vi "SubVI.vi"(0 "AO0波形参数":T1={"波形类型"=2, "幅值"=1.0, "偏置"=0.0, "占空比"=50.0} {"占空比" format="%0.2p"; "偏置" format="%0.2p"; "幅值" format="%0.2p"; "波形类型" items=["正弦波", "三角波", "方波", "锯齿波"]}, 1 "频率比例系数":dbl=9.0 format="%#_13g", 2 "AO8波形参数":cluster{"方向1电压":dbl, "方向2电压":dbl, "方向3电压":dbl}={"方向1电压"=0.5, "方向2电压"=1.0, "方向3电压"=2.0} {"方向3电压" format="%0.2p"; "方向2电压" format="%0.2p"; "方向1电压" format="%0.2p"}, 5 "AO2波形参数":T3={"波形类型"=2, "幅值"=1.0, "偏置"=0.0, "占空比"=50.0, "周期"=0.025} {"占空比" format="%0.2p"; "偏置" format="%0.2p"; "周期" format="%0.2p"; "幅值" format="%0.2p"; "波形类型" items=["正弦波", "三角波", "方波", "锯齿波"]}, 7 "AO4波形参数":T2={"扫描范围(μm)"=10.0, "步长(μm)"=1.0, "转换系数(V/μm)"=0.5, "等待时间(ms)"=3.0} {"等待时间(ms)" format="%0.2p"; "转换系数(V/μm)" format="%0.2p"; "步长(μm)" format="%0.2p"; "扫描范围(μm)" format="%0.2p"}, 9 "AO6波形参数":T1={"波形类型"=2, "幅值"=1.0, "偏置"=0.0, "占空比"=50.0} {"占空比" format="%0.2p"; "偏置" format="%0.2p"; "幅值" format="%0.2p"; "波形类型" items=["正弦波", "三角波", "方波", "锯齿波"]}, 11 "Error in":errorcluster caption="错误输入（无错误）", 12 "采样率":dbl=10000.0) -> (4 "AO0":waveform(dbl)(graph), 6 "AO2":waveform(dbl)(graph), 8 "AO4":waveform(dbl)(graph), 10 "AO6":waveform(dbl)(graph), 13 "AO8":waveform(dbl)(graph), 14 "采样数":dbl=1000.0, 15 "Error out":errorcluster caption="错误输出")   [LabVIEW 2017]
uses:
  <vilib>/measure/NI_MABase.lvlib
  <vilib>/Analysis/NI_AALBase.lvlib
  <vilib>/Analysis/baseanly.llb/Mean (DBL).vi
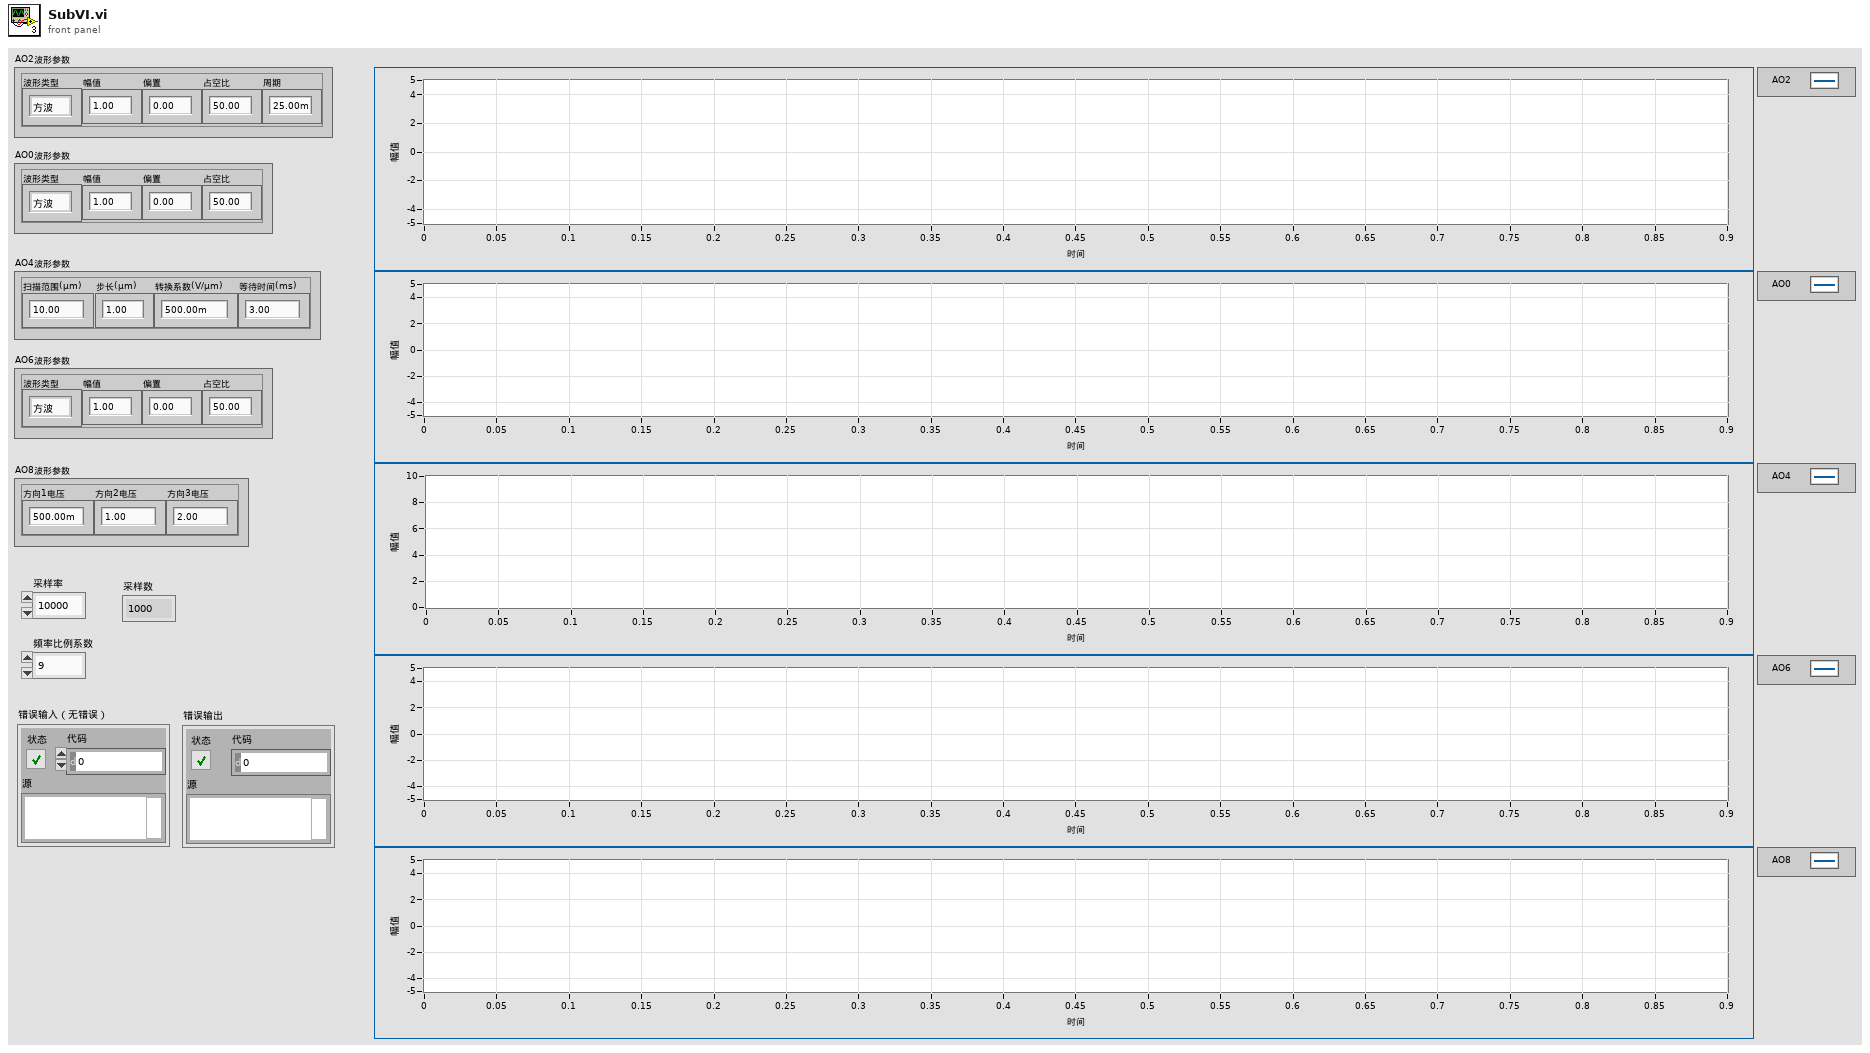
[diagram p1: front panel]
types:
  T1 = cluster{"波形类型":u16, "幅值":dbl, "偏置":dbl, "占空比":dbl}
  T2 = cluster{"扫描范围(μm)":dbl, "步长(μm)":dbl, "转换系数(V/μm)":dbl, "等待时间(ms)":dbl}
  T3 = cluster{"波形类型":u16, "幅值":dbl, "偏置":dbl, "占空比":dbl, "周期":dbl}
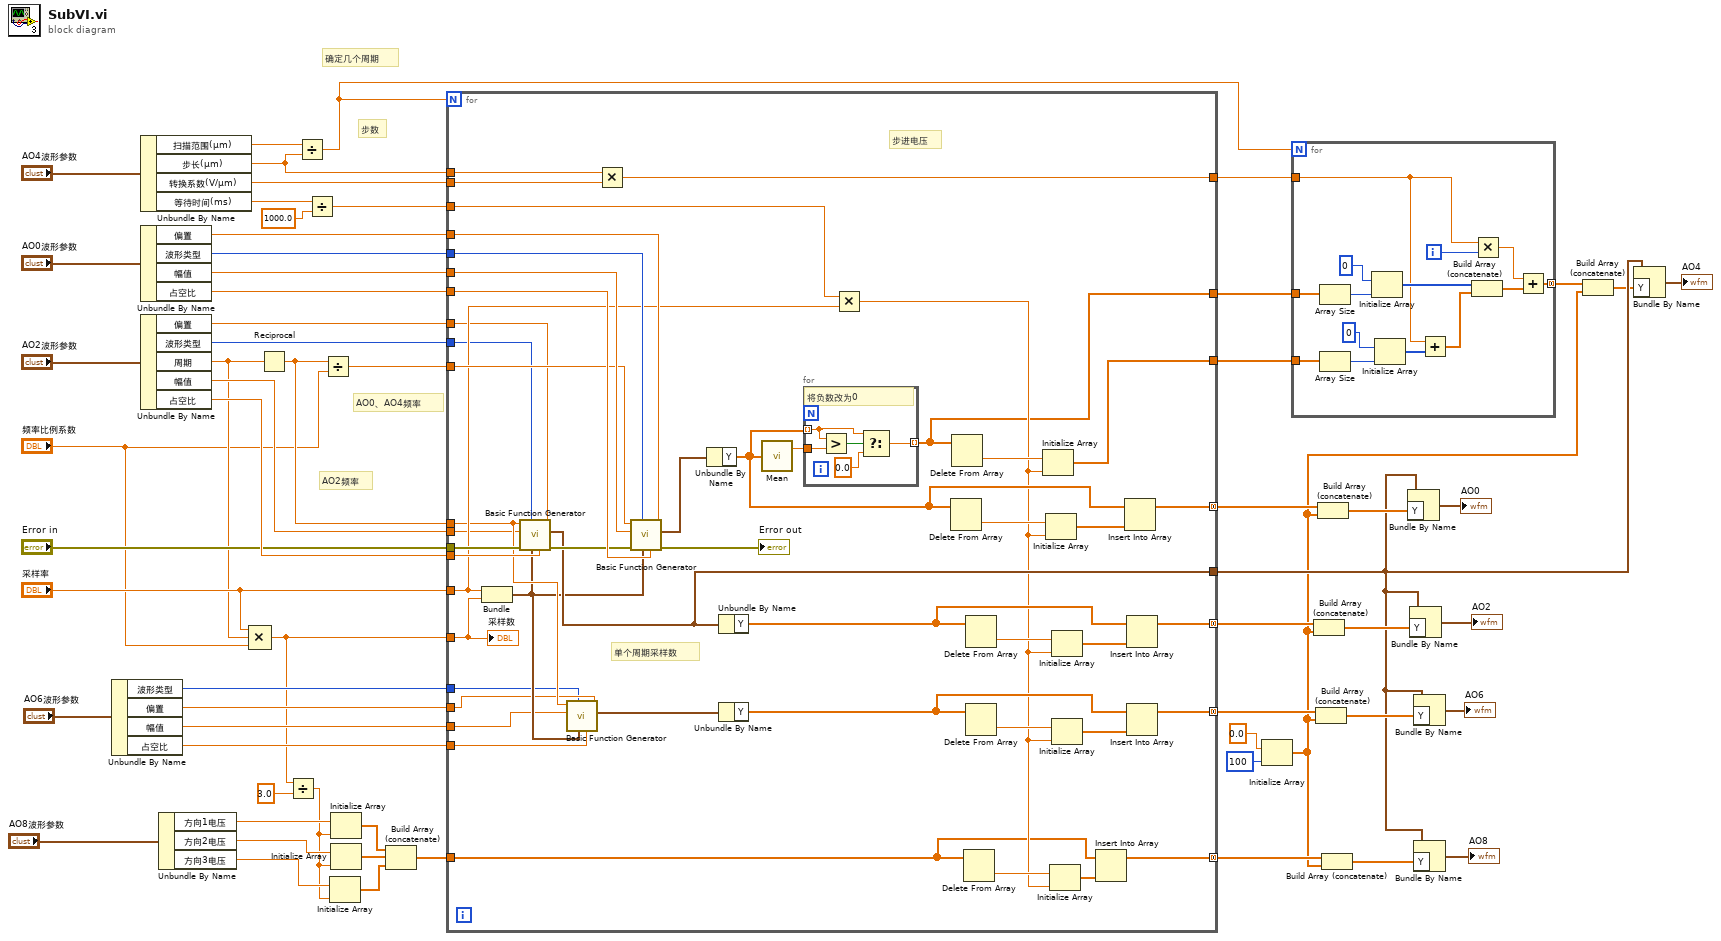
[diagram p0: block diagram]
diagram:
  # "步数"
  # "AO2频率"
  # "AO0、AO4频率"
  # "确定几个周期"
  n1 = Unbundle By Name("AO6波形参数") -> ("波形类型"=w33:u16, "偏置"=w34:dbl, "幅值"=w35:dbl, "占空比"=w36:dbl)
  n2 = Unbundle By Name("AO4波形参数") -> ("扫描范围(μm)"=w49:dbl, "步长(μm)"=w50:dbl, "转换系数(V/μm)"=w51:dbl, "等待时间(ms)"=w46:dbl)
  n3 = Unbundle By Name("AO0波形参数") -> ("偏置"=w57:dbl, "波形类型"=w58:u16, "幅值"=w59:dbl, "占空比"=w62:dbl)
  n4 = Unbundle By Name("AO2波形参数") -> ("偏置"=w56:dbl, "波形类型"=w55:u16, "周期"=w43:dbl, "幅值"=w54:dbl, "占空比"=w61:dbl)
  n5 = Unbundle By Name("AO8波形参数") -> ("方向1电压"=w27:dbl, "方向2电压"=w26:dbl, "方向3电压"=w25:dbl)
  n6 = Compound Arithmetic op=MULTIPLY("采样率", w43, "频率比例系数") -> (w20:dbl)
  n7 = Reciprocal(x=w43) -> (1/x=w44:dbl)
  n8 = Divide(x=w20, y=3.0) -> (x/y=w24:dbl)
  n9 = Divide(x=w49, y=w50) -> (x/y=w16:dbl)
  n10 = Divide(x=w46, y=1000.0) -> (x/y=w41:dbl)
  n11 = Divide(x=w44, y="频率比例系数") -> (x/y=w48:dbl)
  n12 = Initialize Array(w25, w24) -> (w21:dbl[])
  n13 = Initialize Array(w27, w24) -> (w22:dbl[])
  n14 = Initialize Array(w26, w24) -> (w23:dbl[])
  n15 = Build Array (concatenate)(w22, w23, w21) -> (w19:dbl[])
  n16 = for {
    N: w16 -> [_]
    tunnel: w62 -> [w110]
    tunnel: w61 -> [w109]
    tunnel: w59 -> [w106]
    tunnel: w58 -> [w105]
    tunnel: w57 -> [w104]
    tunnel: w56 -> [w82]
    tunnel: w55 -> [w83]
    tunnel: w54 -> [w80]
    tunnel: "Error in" -> [w103]
    tunnel: w51 -> [w102]
    tunnel: [w101] -> w32
    tunnel: w50 -> [w98]
    tunnel: w48 -> [w97]
    tunnel: w20 -> [w96]
    tunnel: "采样率" -> [w95]
    tunnel: w44 -> [w81]
    tunnel: w41 -> [w87]
    tunnel: [w86] -> w8 mode=concatenating
    tunnel: [w85] -> w6 mode=concatenating
    tunnel: [w84] -> w4
    tunnel: w36 -> [w78]
    tunnel: [w73] -> w12 mode=concatenating
    tunnel: w35 -> [w72]
    tunnel: w34 -> [w71]
    tunnel: w33 -> [w70]
    tunnel: w19 -> [w66]
    tunnel: [w65] -> w10 mode=concatenating
    tunnel: [w63] -> w18
    tunnel: [w64] -> w17
    # "步进电压"
    # "单个周期采样数"
    n17 = Bundle("采样率"=w95, w96) -> (w79:cluster{"采样率":dbl, dbl})  [unwired: 1 in]
    n18 = call <vilib>:"Basic Function Generator.vi"("offset"=w82, "square wave duty cycle (%)"=w109, "sampling info"=w79, "signal type"=w83, "error in (no error)"=w103, "amplitude"=w80, "frequency"=w81) -> ("error out"=w107:errorcluster, "signal out"=w84:waveform(dbl))  [unwired: 2 in, 1 out]
    n19 = call <vilib>:"Basic Function Generator.vi"("offset"=w71, "square wave duty cycle (%)"=w78, "sampling info"=w79, "signal type"=w70, "amplitude"=w72, "frequency"=w81) -> ("signal out"=w74:waveform(dbl))  [unwired: 3 in, 2 out]
    n20 = Multiply(x=w98, y=w102) -> (x*y=w101:dbl)
    n21 = call <vilib>:"Basic Function Generator.vi"("offset"=w104, "square wave duty cycle (%)"=w110, "sampling info"=w79, "signal type"=w105, "error in (no error)"=w107, "amplitude"=w106, "frequency"=w97) -> ("error out"=→"Error out":errorcluster, "signal out"=w99:waveform(dbl))  [unwired: 2 in, 1 out]
    n22 = Unbundle By Name(w99) -> ("Y"=w88:dbl[])
    n23 = Unbundle By Name(w84) -> ("Y"=w90:dbl[])
    n24 = Unbundle By Name(w74) -> ("Y"=w77:dbl[])
    n25 = call-poly <vilib>:"Mean.vi"("X"=w88) -> ("mean"=w100:dbl)  [unwired: 1 out]
    n26 = for {
      tunnel: w100 -> [w115]
      tunnel: w88 -> [w113] mode=indexing
      tunnel: [w111] -> w64 mode=indexing
      # "将负数改为0"
      n27 = Greater?(x=w113, y=w115) -> (0:w114:bool)
      n28 = Select(t=w113, s=w114, f=0.0) -> (s? t:f=w111:dbl)
    }
    n29 = Multiply(x=w87, y=w95) -> (x*y=w67:dbl)
    n30 = Delete From Array(array=w88) -> (deleted portion=w93:dbl)  [unwired: 2 in, 1 out]
    n31 = Delete From Array(array=w64) -> (deleted portion=w94:dbl)  [unwired: 2 in, 1 out]
    n32 = Delete From Array(array=w66) -> (deleted portion=w69:dbl)  [unwired: 2 in, 1 out]
    n33 = Delete From Array(array=w90) -> (deleted portion=w92:dbl)  [unwired: 2 in, 1 out]
    n34 = Delete From Array(array=w77) -> (deleted portion=w75:dbl)  [unwired: 2 in, 1 out]
    n35 = Initialize Array(w94, w67) -> (w63:dbl[])
    n36 = Initialize Array(w93, w67) -> (w89:dbl[])
    n37 = Initialize Array(w69, w67) -> (w68:dbl[])
    n38 = Initialize Array(w92, w67) -> (w91:dbl[])
    n39 = Initialize Array(w75, w67) -> (w76:dbl[])
    n40 = Insert Into Array(array=w66, new element=w68) -> (w65:dbl[])  [unwired: 1 in]
    n41 = Insert Into Array(array=w88, new element=w89) -> (w85:dbl[])  [unwired: 1 in]
    n42 = Insert Into Array(array=w90, new element=w91) -> (w86:dbl[])  [unwired: 1 in]
    n43 = Insert Into Array(array=w77, new element=w76) -> (w73:dbl[])  [unwired: 1 in]
    "采样数" <- w96
  }
  n44 = Initialize Array(0.0 ("元素"), 100 ("维数大小")) -> (w2:dbl[])
  n45 = for {
    N: w16 -> [_]
    tunnel: w32 -> [w119]
    tunnel: w18 -> [w124]
    tunnel: w17 -> [w129]
    tunnel: [w116] -> w3 mode=concatenating
    i -> [w118]
    n46 = Array Size(array=w129) -> (size(s)=w128:i32)
    n47 = Array Size(array=w124) -> (size(s)=w123:i32)
    n48 = Initialize Array(0 ("元素"), w128) -> (w126:i32[])
    n49 = Initialize Array(0 ("元素"), w123) -> (w122:i32[])
    n50 = Add(x=w119, y=w122) -> (x+y=w121:dbl[])
    n51 = Build Array (concatenate)(w126, w121) -> (w120:dbl[])
    n52 = Multiply(x=w119, y=w118) -> (x*y=w117:dbl)
    n53 = Add(x=w117, y=w120) -> (x+y=w116:dbl[])
  }
  n54 = Build Array (concatenate)(w8, w2) -> (w7:dbl[])
  n55 = Build Array (concatenate)(w12, w2) -> (w11:dbl[])
  n56 = Build Array (concatenate)(w6, w2) -> (w5:dbl[])
  n57 = Build Array (concatenate)(w10, w2) -> (w9:dbl[])
  n58 = Bundle By Name(cluster=w4, "Y"=w5) -> (→"AO0":waveform(dbl))
  n59 = Bundle By Name(cluster=w4, "Y"=w7) -> (→"AO2":waveform(dbl))
  n60 = Bundle By Name(cluster=w4, "Y"=w11) -> (→"AO6":waveform(dbl))
  n61 = Bundle By Name(cluster=w4, "Y"=w9) -> (→"AO8":waveform(dbl))
  n62 = Build Array (concatenate)(w3, w2) -> (w1:dbl[])
  n63 = Bundle By Name(cluster=w4, "Y"=w1) -> (→"AO4":waveform(dbl))
